vi "Unreserve (Poly).vi"   [LabVIEW 2020, in "Measurement Service Helpers.lvlib"]
doc: "Unreserves the sessions based on the given session information."
uses:
  Measurement Service Helpers.lvlib
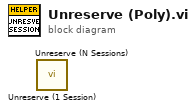
[diagram p0: block diagram]
diagram:
  n1 = call "Unreserve (1 Session).vi"() -> ()  [unwired: 11 in, 1 out]
  n2 = call "Unreserve (N Sessions).vi"() -> ()  [unwired: 11 in, 1 out]
